vi "ComError.vi"() -> ()   [LabVIEW 2016]
panel:
  in  "退出":bool
  out "String":string
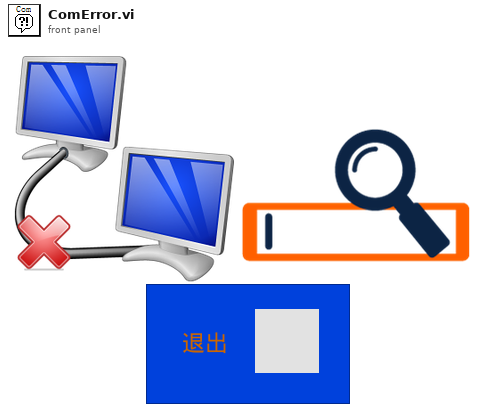
[diagram p1: front panel]
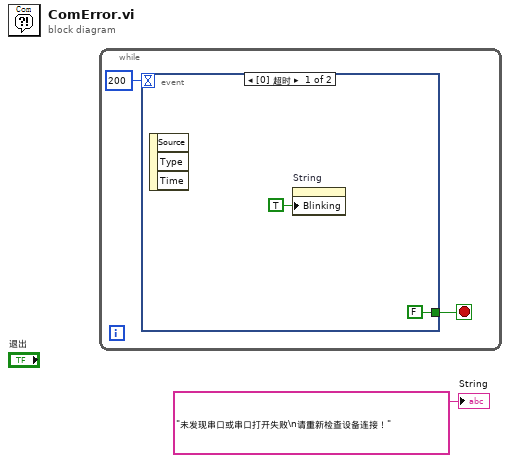
[diagram p0: block diagram]
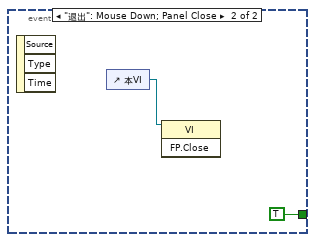
[diagram p2: hidden frame]
diagram:
  n1 = while {
    stop <- w2 stop-if-true
    n2 = event shown="[0] 超时" {
      selector: _ -> [_ _]
      dyn-events: _ -> [_ _]
      timeout: 200 -> [_ _]
      tunnel: [FALSE TRUE] -> w2
      event Timeout {
        n3 = event-data() -> ()  [unwired: 1 in, 3 out]
        n4 = property on="String" class="Str"("Blinking"=TRUE) -> ()  [unwired: 2 in, 2 out]
      }
      event "退出": Mouse Down; Panel Close {
        n5 = event-data() -> ()  [unwired: 1 in, 3 out]
        n6 = control-ref of="本VI"() -> (w7:refnum<vi>)
        n7 = invoke class="VI" method="FP.Close"(reference=w7) -> ()  [unwired: 2 in, 3 out]
      }
    }
  }
  "String" <- "未发现串口或串口打开失败\n请重新检查设备连接！" ("String")
